vi "Fix BDPW Checksum.vi"(8 "error in (no error)":errorcluster, 9 "Terminal Counts":T1, 10 "Only fix 3rd hash (F)":bool, 11 "Resources":T2[](array[typedef])) -> (0 "error out":errorcluster, 3 "Resources out":T2[](array[typedef]))   [LabVIEW 2026, in "VILab.lvlib"]
uses:
  VILab.lvlib
  CTLs/Resource.ctl
  CTLs/Terminal Counts.ctl
  Find Resource by Type (String).vi
  <userlib>/_OpenG.lib/md5/md5.llb/MD5 Message Digest (Binary String)__ogtk.vi
panel:
  # "Thank you Thomas Zeugner! You saved me the trouble of figuring out how this checksum works. :)\nAdapted from https://github.com/tomsoftware/VI-Explorer/blob/master/php/clBDPW.php"
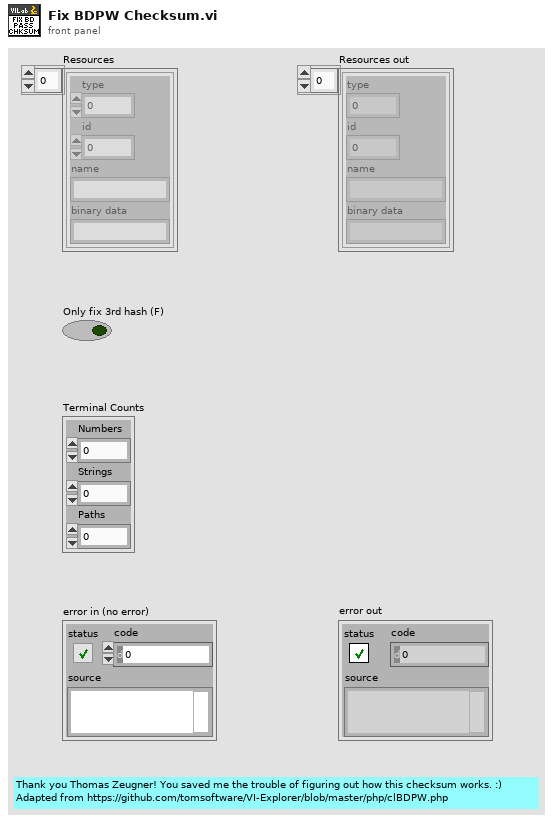
[diagram p1: front panel]
types:
  T1 = typedef "VILab.lvlib/Terminal Counts.ctl" = cluster{"Numbers":u32, "Strings":u32, "Paths":u32}
  T2 = typedef "VILab.lvlib/Resource.ctl" = cluster{"type":u32, "id":i32, "name":string, "binary data":string}
  T3 = enum16{"big-endian, network order", "native, host order", "little-endian"}
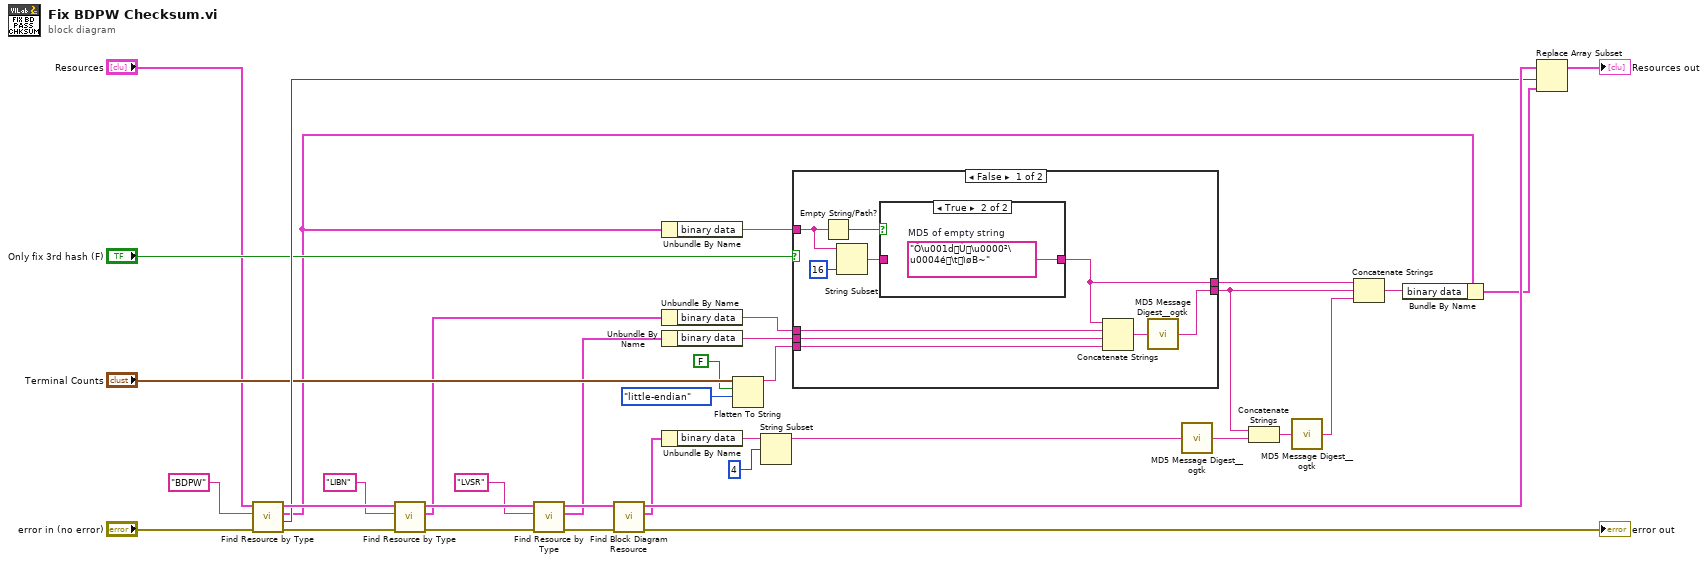
[diagram p0: block diagram]
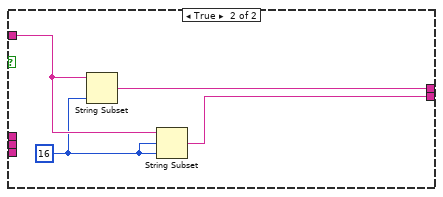
[diagram p3: hidden frame]
diagram:
  n1 = call-poly "Find Resource by Type.vi"("error in (no error)"="error in (no error)", "Resource Type"="BDPW", "Resources"="Resources") -> ("error out"=w5:errorcluster, "Index"=w22:i32, "Resource"=w11:T2, "Resources out"=w37:T2[])  [unwired: 4 in, 1 out]
  n2 = call-poly "Find Resource by Type.vi"("error in (no error)"=w5, "Resource Type"="LIBN", "Resources"=w37) -> ("error out"=w4:errorcluster, "Resource"=w10:T2, "Resources out"=w36:T2[])  [unwired: 4 in, 2 out]
  n3 = call-poly "Find Resource by Type.vi"("error in (no error)"=w4, "Resource Type"="LVSR", "Resources"=w36) -> ("error out"=w3:errorcluster, "Resource"=w8:T2, "Resources out"=w9:T2[])  [unwired: 4 in, 2 out]
  n4 = call "Find Block Diagram Resource.vi"("error in (no error)"=w3, "Resources"=w9) -> ("error out"=→"error out":errorcluster, "Resource"=w6:T2, "Resources out"=w35:T2[])  [unwired: 5 in, 2 out]
  n5 = Unbundle By Name(w11) -> ("binary data"=w18:string)
  n6 = Unbundle By Name(w10) -> ("binary data"=w33:string)
  n7 = Unbundle By Name(w8) -> ("binary data"=w32:string)
  n8 = Unbundle By Name(w6) -> ("binary data"=w26:string)
  n9 = Flatten To String(anything="Terminal Counts", prepend array or string size? (T)=FALSE, byte order (0:big-endian, network order)=T3."little-endian") -> (data string=w14:string)  [unwired: 1 in, 2 out]
  n10 = String Subset(string=w26, offset (0)=4) -> (substring=w24:string)  [unwired: 1 in]
  n11 = case shown="False" "Only fix 3rd hash (F)" {
    tunnel: w33 -> [w46 _]
    tunnel: w32 -> [w45 _]
    tunnel: w14 -> [w43 _]
    tunnel: [w42 w50] -> w17
    tunnel: [w41 w51] -> w19
    tunnel: w18 -> [w39 w53]
    frame False {
      n12 = Empty String/Path?(string/path=w39) -> (empty?=w38:bool)
      n13 = String Subset(string=w39, length (rest)=16 ("length (rest)")) -> (substring=w40:string)  [unwired: 1 in]
      n14 = case shown="True" w38 {
        tunnel: [w48 w49] -> w41
        tunnel: w40 -> [w48 _]
        frame False {
        }
        frame True {
          w49 = "Ô\u001dÙ\u0000²\u0004é\tìøB~"  # MD5 of empty string
        }
      }
      n15 = Concatenate Strings(w41, w46, w45, w43) -> (w44:string)
      n16 = call-poly <userlib>:"MD5 Message Digest__ogtk.vi"("Message"=w44) -> ("MD5 Message Digest"=w42:string)
    }
    frame True {
      w52 = 16 ("length (rest)")
      n17 = String Subset(string=w53, length (rest)=w52) -> (substring=w51:string)  [unwired: 1 in]
      n18 = String Subset(string=w53, offset (0)=w52, length (rest)=w52) -> (substring=w50:string)
    }
  }
  n19 = call-poly <userlib>:"MD5 Message Digest__ogtk.vi"("Message"=w24) -> ("MD5 Message Digest"=w25:string)
  n20 = Concatenate Strings(w17, w25) -> (w28:string)
  n21 = call-poly <userlib>:"MD5 Message Digest__ogtk.vi"("Message"=w28) -> ("MD5 Message Digest"=w27:string)
  n22 = Concatenate Strings(w19, w17, w27) -> (w31:string)
  n23 = Bundle By Name(cluster=w11, "binary data"=w31) -> (w30:T2)
  n24 = Replace Array Subset(array=w35, new element=w30, index=w22) -> (→"Resources out":T2[])
